vi "CreateProduct.vi"(8 "Error In":errorcluster, 11 "reference in":refnum<class "SUVCarFactory.lvclass">) -> (0 "Error Out":errorcluster, 2 "ICarProduct":refnum<class "ICarProduct.lvclass">, 3 "reference out":refnum<class "SUVCarFactory.lvclass">)   [LabVIEW 2024, in "SUVCarFactory.lvclass"]
uses:
  SUVCarFactory.lvclass
  SUVCarFactory.lvclass/SUVCarFactory.ctl
  SUV/SUV.lvclass
  C:/Users/burakkorkmaz/Desktop/Leveling/labview-design-patterns/Factory Method Pattern/Labview/SUV/SUV.lvclass
  C:/Users/burakkorkmaz/Desktop/Leveling/labview-design-patterns/Factory Method Pattern/Labview/ICarProduct/ICarProduct.lvclass
  ICarProduct/ICarProduct.lvclass
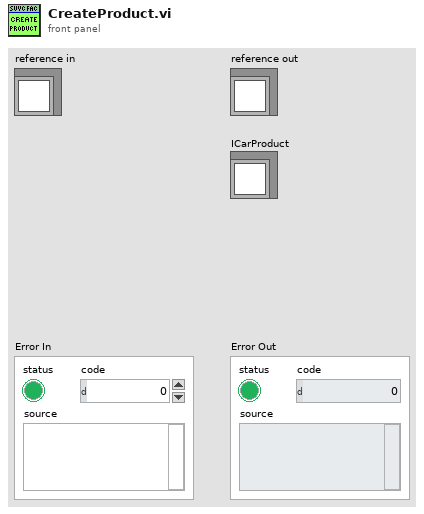
[diagram p1: front panel]
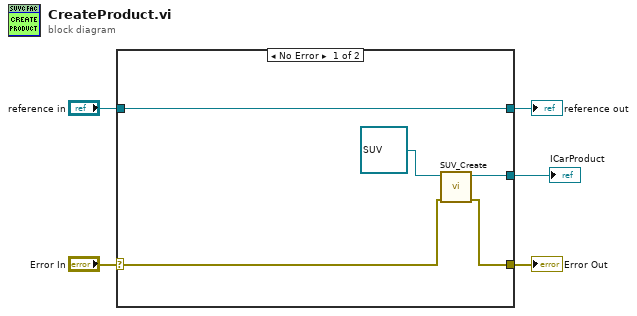
[diagram p0: block diagram]
diagram:
  n1 = case shown="No Error" "Error In" {
    selector: "Error In" -> [w9 w12]
    tunnel: [w8 w12] -> w4
    tunnel: [w10 w11] -> w2
    tunnel: "reference in" -> [w10 w11]
    tunnel: [w6 _] -> w1
    frame No Error {
      n2 = call "SUV_Create.vi"("Error In"=w9, "reference in"=refnum<class "SUV.lvclass"> refnum ("SUV")) -> ("Error Out"=w8:errorcluster, "reference out"=w6:refnum<class "SUV.lvclass">)  [unwired: 8 in]
    }
    frame Error {
    }
  }
  "Error Out" <- w4
  "reference out" <- w2
  "ICarProduct" <- w1
